vi "Module Naming Rules.vi"() -> ()   [LabVIEW 2014]
uses:
  user.lib/_NEVSTOP/Communicable State Machine(CSM)/Communicable State Machine.lvlib
panel:
  out "error 7":errorcluster={"status"=TRUE, "code"=-1, "source"="\"^module\" is not a valid name."}
  out "error 6":errorcluster={"status"=TRUE, "code"=-1, "source"="\"module&name\" is not a valid name."}
  out "error 5":errorcluster
  out "error 4":errorcluster
  out "error 3":errorcluster
  out "error 2":errorcluster
  out "error 1":errorcluster
  out "error 0":errorcluster
  in  "Module Name 7":string="^module"
  in  "Module Name 6":string="module&name"
  in  "Module Name 5":string="module-name"
  in  "Module Name 4":string="module_name"
  in  "Module Name 3":string="Module#"
  in  "Module Name 2":string="Group:Module"
  in  "Module Name 1":string="module name"
  in  "Module Name 0":string="Module "
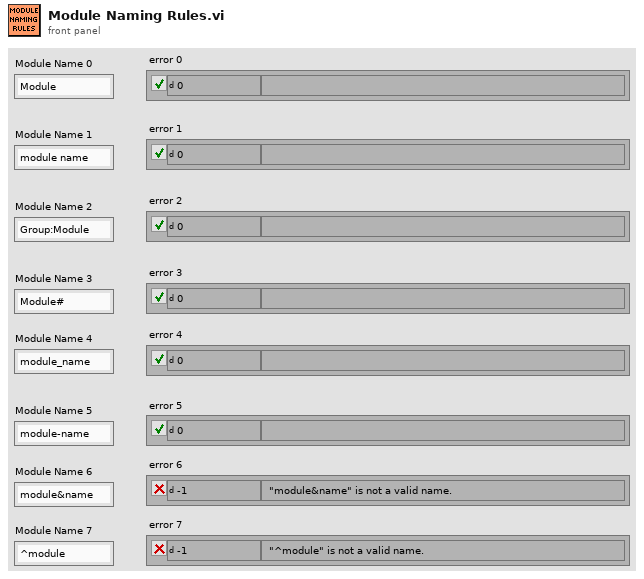
[diagram p1: front panel]
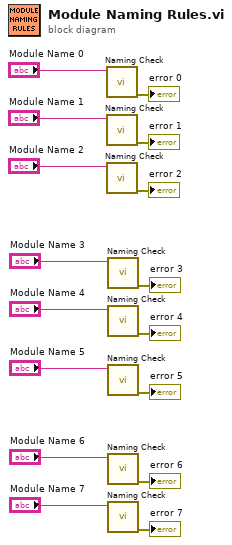
[diagram p0: block diagram]
diagram:
  n1 = call "Naming Check.vi"("Name(\"\" to use uuid)"="Module Name 0") -> ("error out"=→"error 0":errorcluster)  [unwired: 9 in, 1 out]
  n2 = call "Naming Check.vi"("Name(\"\" to use uuid)"="Module Name 1") -> ("error out"=→"error 1":errorcluster)  [unwired: 9 in, 1 out]
  n3 = call "Naming Check.vi"("Name(\"\" to use uuid)"="Module Name 2") -> ("error out"=→"error 2":errorcluster)  [unwired: 9 in, 1 out]
  n4 = call "Naming Check.vi"("Name(\"\" to use uuid)"="Module Name 3") -> ("error out"=→"error 3":errorcluster)  [unwired: 9 in, 1 out]
  n5 = call "Naming Check.vi"("Name(\"\" to use uuid)"="Module Name 4") -> ("error out"=→"error 4":errorcluster)  [unwired: 9 in, 1 out]
  n6 = call "Naming Check.vi"("Name(\"\" to use uuid)"="Module Name 5") -> ("error out"=→"error 5":errorcluster)  [unwired: 9 in, 1 out]
  n7 = call "Naming Check.vi"("Name(\"\" to use uuid)"="Module Name 6") -> ("error out"=→"error 6":errorcluster)  [unwired: 9 in, 1 out]
  n8 = call "Naming Check.vi"("Name(\"\" to use uuid)"="Module Name 7") -> ("error out"=→"error 7":errorcluster)  [unwired: 9 in, 1 out]
